vi "CHP Configure.vi"(0 "Instrument Handle In":refnum<k21>, 5 "CHP Config":T1={"Noise Comp Enabled"=0, "Spectrum Power Units"=9, "Integration Bandwidth (Hz)"=1000000.0, "VBW Auto"=1, "VBW (Hz)"=30000.0, "VBW to RBW Ratio"=3.0, "Span (Hz)"=1000000.0, "Sweep Time Interval (s)"=0.001, "Sweep Time Auto"=1, "RBW Filter Type"=1, "RBW (Hz)"=10000.0, "RBW Auto"=1, "Averaging Enabled"=0, "Averaging Count"=10, "Averaging Type"=0, "Measurement Interval (s)"=0.0001, "Preamp Enabled"=0, "Preselector Enabled"=0} {"Preselector Enabled" items=["Disabled", "Enabled"]; "Preamp Enabled" items=["Disabled"=0, "Enabled"=1, "Automatic"=3]; "Measurement Interval (s)" format="%.3p"; "Averaging Type" items=["RMS", "Log", "Scalar", "Max", "Min"]; "Averaging Enabled" items=["False", "True"]; "RBW Auto" items=["False", "True"]; "RBW (Hz)" format="%.3p"; "RBW Filter Type" items=["FFT Based", "Gaussian", "Flat"]; "Sweep Time Auto" items=["False", "True"]; "Sweep Time Interval (s)" format="%.2p"; "Span (Hz)" format="%.3p"; "VBW to RBW Ratio" format="%#.6f"; "VBW (Hz)" format="%.3p"; "VBW Auto" items=["False", "True"]; "Integration Bandwidth (Hz)" format="%.3p"; "Spectrum Power Units" items=["dBm", "dBm/Hz", "dBW", "dBV", "dBmV", "dBuV", "W", "Volts", "Volts Squared", "Reference Level Units"]; "Noise Comp Enabled" items=["False", "True"]}, 11 "error in (no error)":errorcluster) -> (4 "Instrument Handle Out":refnum<k21>, 15 "error out":errorcluster)   [LabVIEW 2018, in "RFmxSpecAn.lvlib"]
uses:
  RFmxSpecAn.lvlib
  Typedefs/CHP Configuration.ctl
  <vilib>/RFmx/SpecAn/mx/RFmxSpecAn.llb/RFmxSpecAn Select Measurement (Multiple).vi
  <resource>/objmgr/RFmxInstr.rc
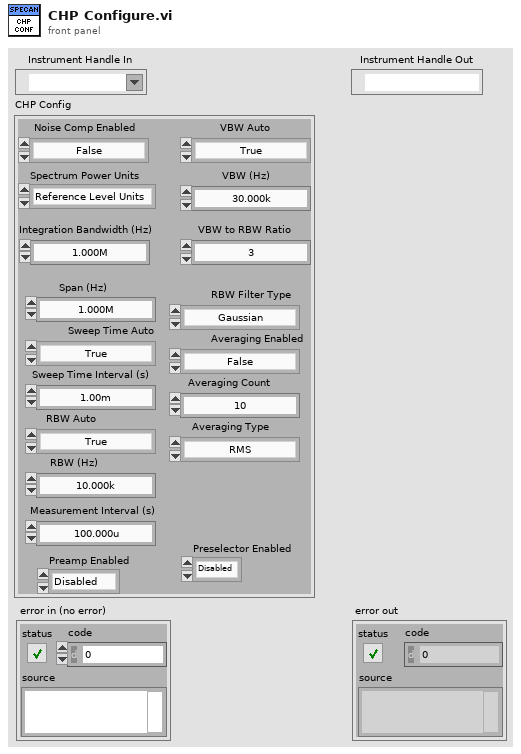
[diagram p1: front panel]
types:
  T1 = typedef "RFmxSpecAn.lvlib/CHP Configuration.ctl" = cluster{"Noise Comp Enabled":i32, "Spectrum Power Units":i32, "Integration Bandwidth (Hz)":dbl, "VBW Auto":i32, "VBW (Hz)":dbl, "VBW to RBW Ratio":dbl, "Span (Hz)":dbl, "Sweep Time Interval (s)":dbl, "Sweep Time Auto":i32, "RBW Filter Type":i32, "RBW (Hz)":dbl, "RBW Auto":i32, "Averaging Enabled":i32, "Averaging Count":i32, "Averaging Type":i32, "Measurement Interval (s)":dbl, "Preamp Enabled":i32, "Preselector Enabled":i32}
  T2 = enum16{"ACP", "CCDF", "CHP", "FCnt", "Harmonics", "OBW", "SEM", "Spectrum", "Spur", "TXP", "AMPM", "DPD", "IQ", "IM", "NF", "PhaseNoise"}[]
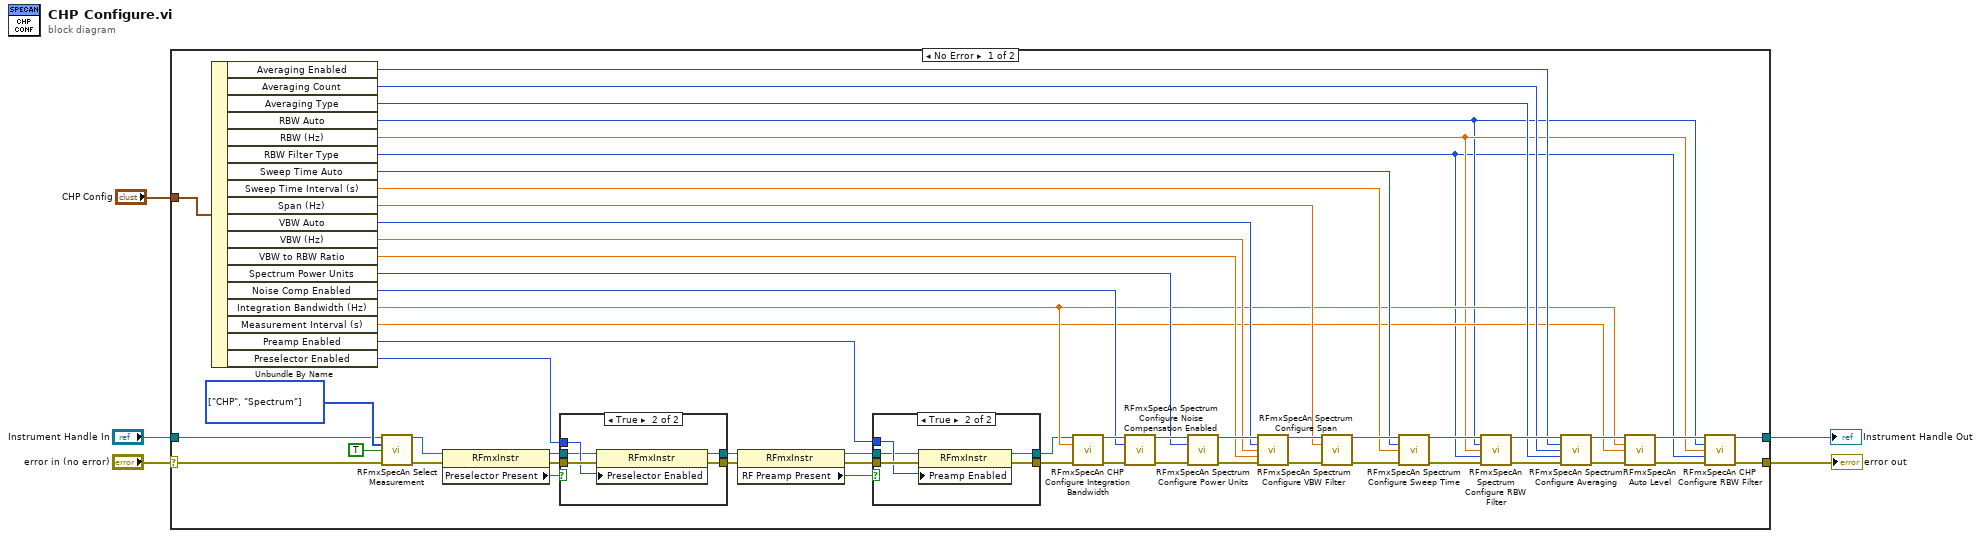
[diagram p0: block diagram]
diagram:
  n1 = case shown="No Error" "error in (no error)" {
    selector: "error in (no error)" -> [w46 w76]
    tunnel: "CHP Config" -> [w52 _]
    tunnel: "Instrument Handle In" -> [w27 w75]
    tunnel: [w10 w75] -> w3
    tunnel: [w9 w76] -> w1
    frame No Error {
      w59 = T2 [enum."CHP", enum."Spectrum"] items=["ACP", "CCDF", "CHP", "FCnt", "Harmonics", "OBW", "SEM", "Spectrum", "Spur", "TXP", "AMPM", "DPD", "IQ", "IM", "NF", "PhaseNoise"]
      n2 = Unbundle By Name(w52) -> ("Averaging Enabled"=w32:i32, "Averaging Count"=w33:i32, "Averaging Type"=w34:i32, "RBW Auto"=w7:i32, "RBW (Hz)"=w8:dbl, "RBW Filter Type"=w6:i32, "Sweep Time Auto"=w35:i32, "Sweep Time Interval (s)"=w36:dbl, "Span (Hz)"=w37:dbl, "VBW Auto"=w51:i32, "VBW (Hz)"=w50:dbl, "VBW to RBW Ratio"=w49:dbl, "Spectrum Power Units"=w48:i32, "Noise Comp Enabled"=w47:i32, "Integration Bandwidth (Hz)"=w29:dbl, "Measurement Interval (s)"=w28:dbl, "Preamp Enabled"=w13:i32, "Preselector Enabled"=w22:i32)
      n3 = call-poly <vilib>:"RFmxSpecAn Select Measurement.vi"("Instrument Handle In"=w27, "Measurements"=w59, "Enable All Traces"=TRUE, "error in (no error)"=w46) -> ("Instrument Handle Out"=w26:refnum<k21>, "error out"=w25:errorcluster)  [unwired: 10 in]
      n4 = property class="RFmxInstr"(reference=w26, error in=w25) -> (reference out=w21:refnum<k21>, error out=w23:errorcluster, "Preselector Present"=w24:bool)
      n5 = case shown="True" w24 {
        tunnel: w23 -> [w61 w67]
        tunnel: w22 -> [_ w66]
        tunnel: w21 -> [w62 w65]
        tunnel: [w61 w64] -> w18
        tunnel: [w62 w63] -> w17
        frame False {
        }
        frame True {
          n6 = property class="RFmxInstr"(reference=w65, error in=w67, "Preselector Enabled"=w66) -> (reference out=w63:refnum<k21>, error out=w64:errorcluster)
        }
      }
      n7 = property class="RFmxInstr"(reference=w17, error in=w18) -> (reference out=w14:refnum<k21>, error out=w15:errorcluster, "RF Preamp Present"=w16:bool)
      n8 = case shown="True" w16 {
        tunnel: w15 -> [w68 w74]
        tunnel: w13 -> [_ w73]
        tunnel: w14 -> [w69 w72]
        tunnel: [w68 w71] -> w20
        tunnel: [w69 w70] -> w19
        frame False {
        }
        frame True {
          n9 = property class="RFmxInstr"(reference=w72, error in=w74, "Preamp Enabled"=w73) -> (reference out=w70:refnum<k21>, error out=w71:errorcluster)
        }
      }
      n10 = call <vilib>:"RFmxSpecAn CHP Configure Integration Bandwidth.vi"("Instrument Handle In"=w19, "Integration Bandwidth (Hz)"=w29, "error in (no error)"=w20) -> ("Instrument Handle Out"=w54:refnum<k21>, "error out"=w53:errorcluster)  [unwired: 11 in]
      n11 = call <vilib>:"RFmxSpecAn Spectrum Configure Noise Compensation Enabled.vi"("Instrument Handle In"=w54, "Spectrum Noise Comp Enabled"=w47, "error in (no error)"=w53) -> ("Instrument Handle Out"=w57:refnum<k21>, "error out"=w58:errorcluster)  [unwired: 11 in]
      n12 = call <vilib>:"RFmxSpecAn Spectrum Configure Power Units.vi"("Instrument Handle In"=w57, "Power Units"=w48, "error in (no error)"=w58) -> ("Instrument Handle Out"=w55:refnum<k21>, "error out"=w56:errorcluster)  [unwired: 11 in]
      n13 = call <vilib>:"RFmxSpecAn Spectrum Configure VBW Filter.vi"("Instrument Handle In"=w55, "VBW Auto"=w51, "VBW (Hz)"=w50, "VBW to RBW Ratio"=w49, "error in (no error)"=w56) -> ("Instrument Handle Out"=w41:refnum<k21>, "error out"=w42:errorcluster)  [unwired: 9 in]
      n14 = call <vilib>:"RFmxSpecAn Spectrum Configure Span.vi"("Instrument Handle In"=w41, "Span (Hz)"=w37, "error in (no error)"=w42) -> ("Instrument Handle Out"=w40:refnum<k21>, "error out"=w43:errorcluster)  [unwired: 11 in]
      n15 = call <vilib>:"RFmxSpecAn Spectrum Configure Sweep Time.vi"("Instrument Handle In"=w40, "Sweep Time Auto"=w35, "Sweep Time Interval (s)"=w36, "error in (no error)"=w43) -> ("Instrument Handle Out"=w39:refnum<k21>, "error out"=w44:errorcluster)  [unwired: 10 in]
      n16 = call <vilib>:"RFmxSpecAn Spectrum Configure RBW Filter.vi"("Instrument Handle In"=w39, "RBW Auto"=w7, "RBW (Hz)"=w8, "RBW Filter Type"=w6, "error in (no error)"=w44) -> ("Instrument Handle Out"=w38:refnum<k21>, "error out"=w45:errorcluster)  [unwired: 9 in]
      n17 = call <vilib>:"RFmxSpecAn Spectrum Configure Averaging.vi"("Instrument Handle In"=w38, "Averaging Enabled"=w32, "Averaging Count"=w33, "Averaging Type"=w34, "error in (no error)"=w45) -> ("Instrument Handle Out"=w30:refnum<k21>, "error out"=w31:errorcluster)  [unwired: 9 in]
      n18 = call <vilib>:"RFmxSpecAn Auto Level.vi"("Instrument Handle In"=w30, "Bandwidth (Hz)"=w29, "Measurement Interval (s)"=w28, "error in (no error)"=w31) -> ("Instrument Handle Out"=w12:refnum<k21>, "error out"=w11:errorcluster)  [unwired: 9 in, 1 out]
      n19 = call <vilib>:"RFmxSpecAn CHP Configure RBW Filter.vi"("Instrument Handle In"=w12, "RBW Auto"=w7, "RBW (Hz)"=w8, "RBW Filter Type"=w6, "error in (no error)"=w11) -> ("Instrument Handle Out"=w10:refnum<k21>, "error out"=w9:errorcluster)  [unwired: 9 in]
    }
    frame Error {
    }
  }
  "error out" <- w1
  "Instrument Handle Out" <- w3
